vi "test target.vi"(6 "Numeric":dbl, 11 "Class 1.lvclass":refnum<class "Class 1.lvclass">) -> (3 "Class 1.lvclass 2":refnum<class "Class 1.lvclass">)   [LabVIEW 2019]
uses:
  Class 1.lvclass
panel:
  in  "Boolean 3":bool
  in  "data value reference 2":refnum<data-value>
  in  "data value reference":refnum<data-value>
  in  "Boolean 2":bool
  out "Boolean":bool
  out "Numeric 2":dbl
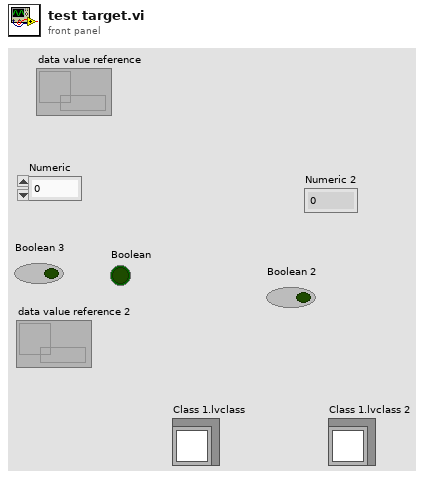
[diagram p1: front panel]
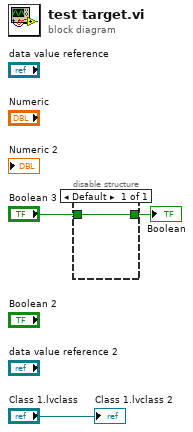
[diagram p0: block diagram]
diagram:
  n1 = disable-structure shown="Default" {
    disable-tunnel: [w4] -> w3
    disable-tunnel: "Boolean 3" -> [w4]
    frame Enabled {
    }
  }
  "Boolean" <- w3
  "Class 1.lvclass 2" <- "Class 1.lvclass"
